vi "Check Voltage Bounds.vi"(0 "channel configuration":T1[](array[typedef]) {"vertical offset" format="%_3p"; "vertical range" format="%_3p"}, 5 "trigger source":u8, 7 "level (V)":dbl, 11 "error in":errorcluster) -> (15 "error out":errorcluster)   [LabVIEW 2021, in "Device Session.lvclass"]
uses:
  Device Session.lvclass
  <instrlib>/HSAI-RIO/Types/v1/Host/Typedefs/Channel Configuration.ctl
  <instrlib>/HSAI-RIO/Types/v1/Host/Typedefs/Coupling.ctl
  <instrlib>/HSAI-RIO/Types/v1/Host/Typedefs/Impedance.ctl
  <instrlib>/HSAI-RIO/Types/v1/Host/Typedefs/Bandwidth.ctl
  <vilib>/Utility/error.llb/Error Cluster From Error Code.vi
  <vilib>/ErrorRing/Error Ring.xnode
  <instrlib>/HSAI-RIO/Types/v1/Host/niHSAI Types v1 Host.lvlib
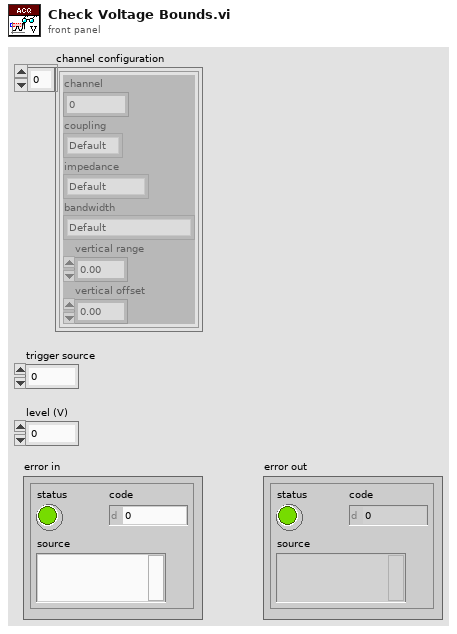
[diagram p1: front panel]
types:
  T1 = typedef "niHSAI Types v1 Host.lvlib/Channel Configuration.ctl" = cluster{"channel":u32, "coupling":T2, "impedance":T3, "bandwidth":T4, "vertical range":dbl, "vertical offset":dbl}
  T2 = typedef "niHSAI Types v1 Host.lvlib/Coupling.ctl" = enum8{"Default", "DC", "AC"}
  T3 = typedef "niHSAI Types v1 Host.lvlib/Impedance.ctl" = enum8{"Default", "1 mega ohm", "50 ohm"}
  T4 = typedef "niHSAI Types v1 Host.lvlib/Bandwidth.ctl" = enum8{"Default", "Full Bandwidth", "Anti-alias Filter", "150 MHz"}
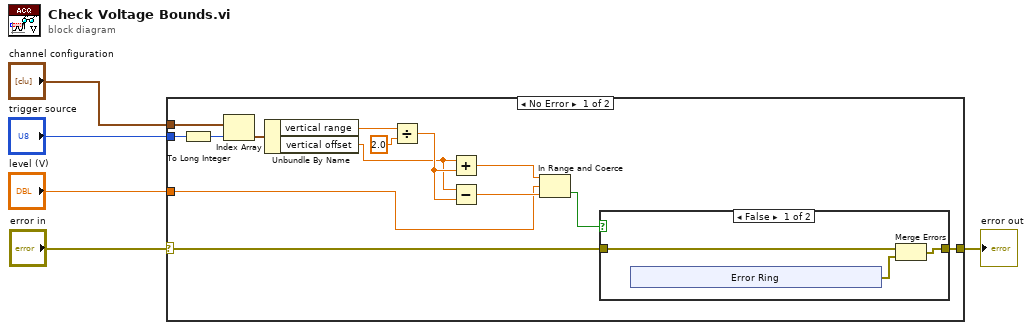
[diagram p0: block diagram]
diagram:
  n1 = case shown="No Error" "error in" {
    selector: "error in" -> [w15 w28]
    tunnel: "channel configuration" -> [w17 _]
    tunnel: "trigger source" -> [w13 _]
    tunnel: "level (V)" -> [w6 _]
    tunnel: [w16 w28] -> w1
    frame No Error {
      n2 = To Long Integer(number=w13) -> (32bit integer=w14:i32)
      n3 = Index Array(array=w17, index=w14) -> (element=w19:T1)
      n4 = Unbundle By Name(w19) -> ("vertical range"=w18:dbl, "vertical offset"=w7:dbl)
      n5 = Divide(x=w18, y=2.0 ("vertical range")) -> (x/y=w11:dbl)
      n6 = Add(x=w7, y=w11) -> (x+y=w10:dbl)
      n7 = Subtract(x=w7, y=w11) -> (x-y=w9:dbl)
      n8 = In Range and Coerce(upper limit=w10, x=w6, lower limit=w9) -> (In Range?=w8:bool)  [unwired: 1 out]
      n9 = case shown="False" w8 {
        tunnel: [w22 w27] -> w16
        tunnel: w15 -> [w20 w27]
        frame False {
          n10 = xnode "Error Ring"() -> ("error out"=w21:errorcluster)
          n11 = Merge Errors(w20, w21) -> (w22:errorcluster)
        }
        frame True {
        }
      }
    }
    frame Error {
    }
  }
  "error out" <- w1
